vi "__Test_LvDataToMemory_NOPTR.vi"() -> ()   [LabVIEW 2019]
uses:
  __cvi/__TEST_CVI_Prj_NOPTR/TEST_DataType.dll
  Memory Data Access.lvlib
panel:
  out "Ret_Cluster":i32
  out "Ret_ArrayWav":u32
  out "Ret_Waveform":u32
  out "Ret_TimeStamp":dbl
  out "Ret_ArrayStr":u32
  out "ByteArray":u8[](array[numeric])
  out "Ret_ArrayDBL":u32
  out "Ret_Path":i32
  out "Ret_Str":i32
  out "Ret_Boolean":u8
  out "Ret_DBL":dbl
  out "Ret_I32":i32
  out "Ret_U32":u32
  in  "Enum":T1(ring)
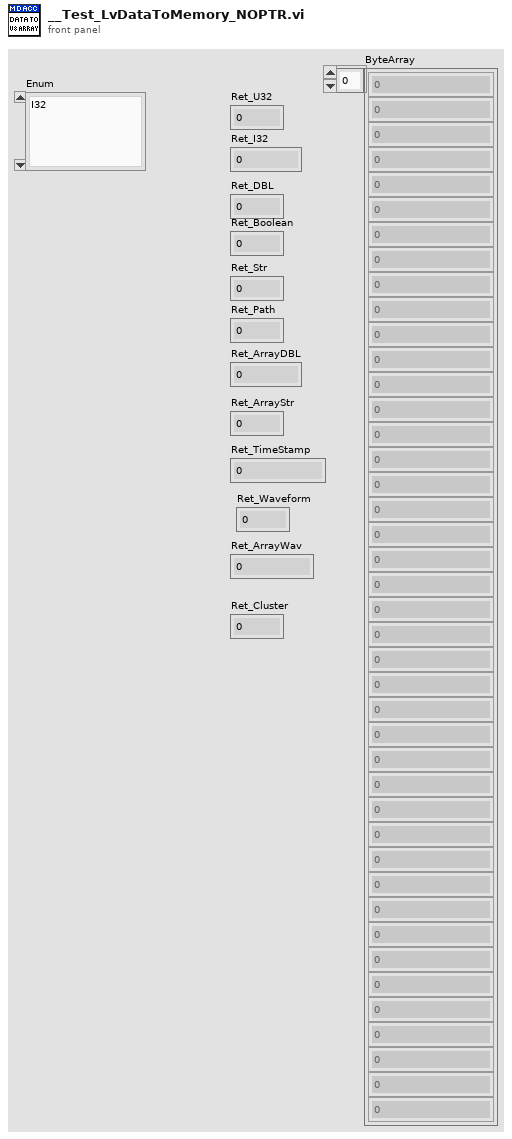
[diagram p1: front panel]
types:
  T1 = enum16{"I32", "U32", "DBL", "String", "Cluster", "Array_Str", "Array_DBL", "Array_Waveform", "Bool", "TimeStamp", "Waveform", "Path"}
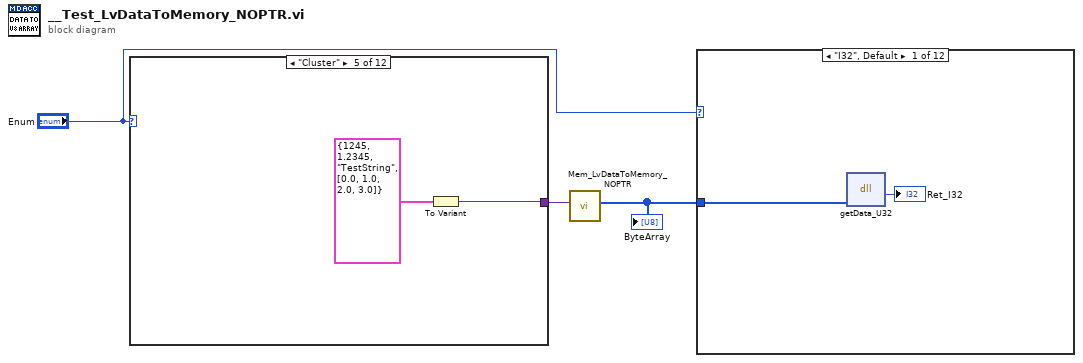
[diagram p0: block diagram]
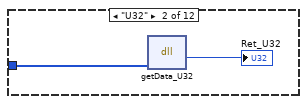
[diagram p2: hidden frame]
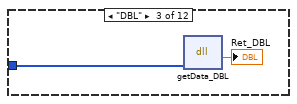
[diagram p3: hidden frame]
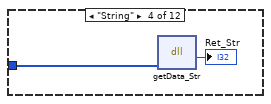
[diagram p4: hidden frame]
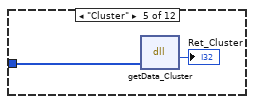
[diagram p5: hidden frame]
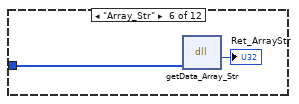
[diagram p6: hidden frame]
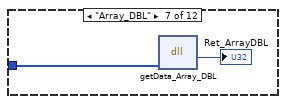
[diagram p7: hidden frame]
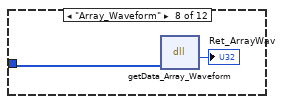
[diagram p8: hidden frame]
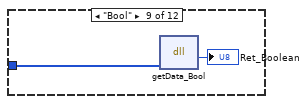
[diagram p9: hidden frame]
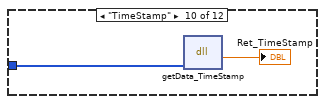
[diagram p10: hidden frame]
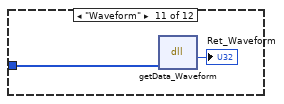
[diagram p11: hidden frame]
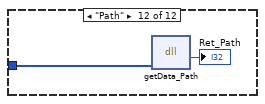
[diagram p12: hidden frame]
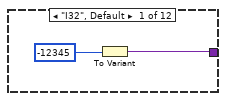
[diagram p13: hidden frame]
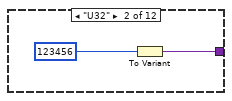
[diagram p14: hidden frame]
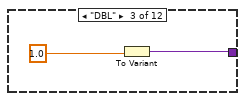
[diagram p15: hidden frame]
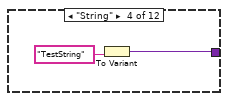
[diagram p16: hidden frame]
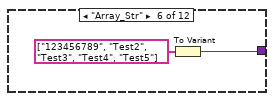
[diagram p17: hidden frame]
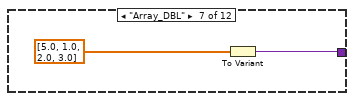
[diagram p18: hidden frame]
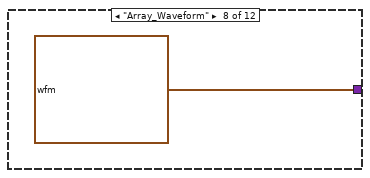
[diagram p19: hidden frame]
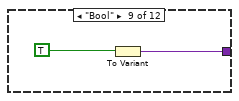
[diagram p20: hidden frame]
diagram:
  n1 = case shown="\"Cluster\"" "Enum" {
    tunnel: [w5 w7 w9 w11 w13 w14 w17 waveform(dbl)[] [{"t0"=timestamp(3705278400 s since 1904-01-01), "dt"=1.0, "Y"=[1.0, 2.0, 3.0]}, {"t0"=timestamp(3705278400 s since 1904-01-01), "dt"=1.0, "Y"=[4.0, 5.0, 6.0, 7.0]}] w20 w22 w24 w26] -> w3
    frame "I32", Default {
      n2 = To Variant(anything=-12345) -> (Variant=w5:variant)
    }
    frame "U32" {
      n3 = To Variant(anything=u32 123456) -> (Variant=w7:variant)
    }
    frame "DBL" {
      n4 = To Variant(anything=1.0) -> (Variant=w9:variant)
    }
    frame "String" {
      n5 = To Variant(anything="TestString") -> (Variant=w11:variant)
    }
    frame "Cluster" {
      n6 = To Variant(anything=cluster{i32, dbl, string, dbl[]} {1245, 1.2345, "TestString", [0.0, 1.0, 2.0, 3.0]}) -> (Variant=w13:variant)
    }
    frame "Array_Str" {
      n7 = To Variant(anything=string[] ["123456789", "Test2", "Test3", "Test4", "Test5"]) -> (Variant=w14:variant)
    }
    frame "Array_DBL" {
      n8 = To Variant(anything=dbl[] [5.0, 1.0, 2.0, 3.0]) -> (Variant=w17:variant)
    }
    frame "Array_Waveform" {
    }
    frame "Bool" {
      n9 = To Variant(anything=TRUE) -> (Variant=w20:variant)
    }
    frame "TimeStamp" {
      w21 = timestamp(3438133200 s since 1904-01-01)
      n10 = To Double Precision Float(number=w21) -> ()  [unwired: 1 out]
      n11 = To Variant(anything=w21) -> (Variant=w22:variant)
    }
    frame "Waveform" {
      n12 = To Variant(anything=waveform(dbl) {"t0"=timestamp(3722126400 s since 1904-01-01), "dt"=1.0, "Y"=[1.0, 2.0, 3.0, 4.0]} ("Waveform")) -> (Variant=w24:variant)
    }
    frame "Path" {
      n13 = To Variant(anything=path "C:/Test/File") -> (Variant=w26:variant)
    }
  }
  n14 = call "Mem_LvDataToMemory_NOPTR.vi"("Payload"=w3) -> ("ByteArray"=w1:u8[])  [unwired: 8 in, 2 out]
  "ByteArray" <- w1
  n15 = case shown="\"I32\", Default" "Enum" {
    tunnel: w1 -> [w28 w30 w32 w34 w36 w38 w40 w42 w44 w46 w48 w50]
    frame "I32", Default {
      n16 = dll-call lib="D:/Workspace/_TEST/Memory-Data-Access/__cvi/__TEST_CVI_Prj_NOPTR/TEST_DataType.dll" fn="getData_U32"("Para"=w28) -> ("return type"=→"Ret_I32":i32)  [unwired: 4 in, 2 out]
    }
    frame "U32" {
      n17 = dll-call lib="D:/Workspace/_TEST/Memory-Data-Access/__cvi/__TEST_CVI_Prj_NOPTR/TEST_DataType.dll" fn="getData_U32"("Para"=w30) -> ("return type"=→"Ret_U32":u32)  [unwired: 4 in, 2 out]
    }
    frame "DBL" {
      n18 = dll-call lib="D:/Workspace/_TEST/Memory-Data-Access/__cvi/__TEST_CVI_Prj_NOPTR/TEST_DataType.dll" fn="getData_DBL"("Para"=w32) -> ("return type"=→"Ret_DBL":dbl)  [unwired: 4 in, 2 out]
    }
    frame "String" {
      n19 = dll-call lib="D:/Workspace/_TEST/Memory-Data-Access/__cvi/__TEST_CVI_Prj_NOPTR/TEST_DataType.dll" fn="getData_Str"("Para"=w34) -> ("return type"=→"Ret_Str":i32)  [unwired: 4 in, 2 out]
    }
    frame "Cluster" {
      n20 = dll-call lib="D:/Workspace/_TEST/Memory-Data-Access/__cvi/__TEST_CVI_Prj_NOPTR/TEST_DataType.dll" fn="getData_Cluster"("Para"=w36) -> ("return type"=→"Ret_Cluster":i32)  [unwired: 4 in, 2 out]
    }
    frame "Array_Str" {
      n21 = dll-call lib="D:/Workspace/_TEST/Memory-Data-Access/__cvi/__TEST_CVI_Prj_NOPTR/TEST_DataType.dll" fn="getData_Array_Str"("Para"=w38) -> ("return type"=→"Ret_ArrayStr":u32)  [unwired: 4 in, 2 out]
    }
    frame "Array_DBL" {
      n22 = dll-call lib="D:/Workspace/_TEST/Memory-Data-Access/__cvi/__TEST_CVI_Prj_NOPTR/TEST_DataType.dll" fn="getData_Array_DBL"("Para"=w40) -> ("return type"=→"Ret_ArrayDBL":u32)  [unwired: 4 in, 2 out]
    }
    frame "Array_Waveform" {
      n23 = dll-call lib="D:/Workspace/_TEST/Memory-Data-Access/__cvi/__TEST_CVI_Prj_NOPTR/TEST_DataType.dll" fn="getData_Array_Waveform"("Para"=w42) -> ("return type"=→"Ret_ArrayWav":u32)  [unwired: 4 in, 2 out]
    }
    frame "Bool" {
      n24 = dll-call lib="D:/Workspace/_TEST/Memory-Data-Access/__cvi/__TEST_CVI_Prj_NOPTR/TEST_DataType.dll" fn="getData_Bool"("Para"=w44) -> ("return type"=→"Ret_Boolean":u8)  [unwired: 4 in, 2 out]
    }
    frame "TimeStamp" {
      n25 = dll-call lib="D:/Workspace/_TEST/Memory-Data-Access/__cvi/__TEST_CVI_Prj_NOPTR/TEST_DataType.dll" fn="getData_TimeStamp"("Para"=w46) -> ("return type"=→"Ret_TimeStamp":dbl)  [unwired: 4 in, 2 out]
    }
    frame "Waveform" {
      n26 = dll-call lib="D:/Workspace/_TEST/Memory-Data-Access/__cvi/__TEST_CVI_Prj_NOPTR/TEST_DataType.dll" fn="getData_Waveform"("Para"=w48) -> ("return type"=→"Ret_Waveform":u32)  [unwired: 4 in, 2 out]
    }
    frame "Path" {
      n27 = dll-call lib="D:/Workspace/_TEST/Memory-Data-Access/__cvi/__TEST_CVI_Prj_NOPTR/TEST_DataType.dll" fn="getData_Path"("Para"=w50) -> ("return type"=→"Ret_Path":i32)  [unwired: 4 in, 2 out]
    }
  }
